vi "convertFloatToCounter.vi"(10 "Numeric":dbl format="%#_11g") -> (2 "Counter Version":u32)   [LabVIEW 2017]
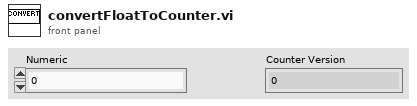
[diagram p1: front panel]
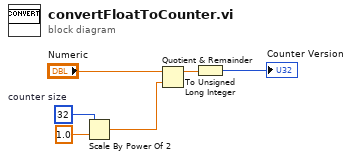
[diagram p0: block diagram]
diagram:
  w4 = i16 32  # counter size
  n1 = Scale By Power Of 2(n=w4, x=1.0) -> (x*2^n=w1:dbl)
  n2 = Quotient & Remainder(x="Numeric", y=w1) -> (x-y*floor(x/y)=w3:dbl)  [unwired: 1 out]
  n3 = To Unsigned Long Integer(number=w3) -> (unsigned 32bit integer=→"Counter Version":u32)
